vi "Graph Sine Array.vi"() -> ()   [LabVIEW 2017]
panel:
  out "Error Out":errorcluster
  in  "Error In":errorcluster
  out "Waveform Array":dbl[](array[numeric])
  out "Graph":dbl[][](graph)
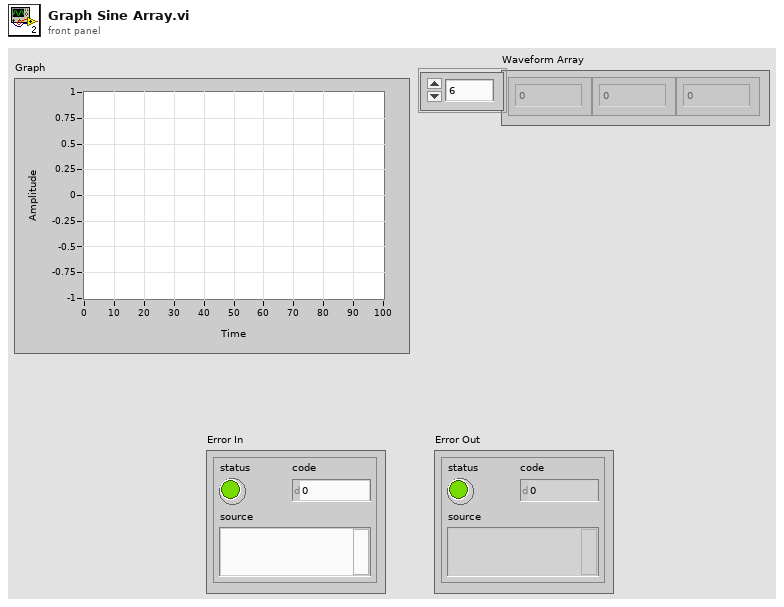
[diagram p1: front panel]
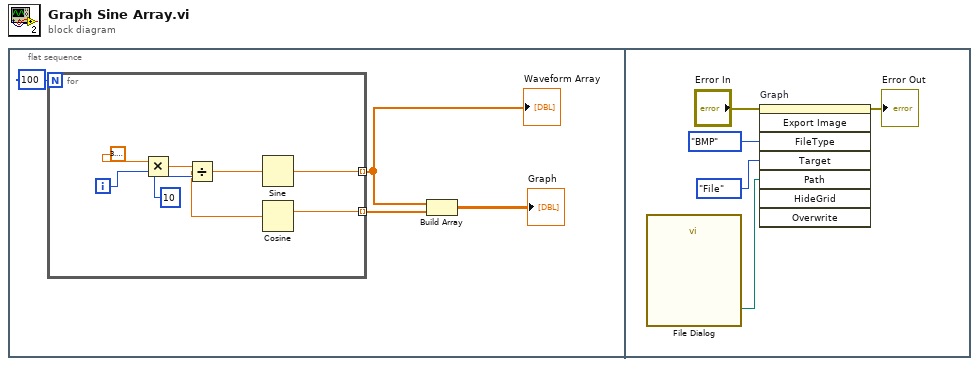
[diagram p0: block diagram]
diagram:
  n1 = flat-sequence {
    frame #0 {
      n2 = for {
        N: 100 -> [_]
        tunnel: [w7] -> w2 mode=indexing
        tunnel: [w5] -> w3 mode=indexing
        i -> [w10]
        n3 = Multiply(x=3.141592653589793, y=w10) -> (x*y=w9:dbl)
        n4 = Divide(x=w9, y=10) -> (x/y=w6:dbl)
        n5 = Sine(x=w6) -> (sin(x)=w7:dbl)
        n6 = Cosine(x=w6) -> (cos(x)=w5:dbl)
      }
      "Waveform Array" <- w2
      n7 = Build Array "Build Array"(w2, w3) -> (→"Graph":dbl[][])
    }
    frame #1 {
      n8 = call "File Dialog"() -> ("selected path"=w16:path)  [unwired: 12 in, 3 out]
      n9 = invoke on="Graph" class="WFGraph (strict)" method="Export Image"(error in="Error In", "FileType"=enum16{"BMP"}."BMP", "Target"=enum16{"File"}."File", "Path"=w16) -> (error out=→"Error Out":errorcluster)  [unwired: 4 in, 7 out]
    }
  }
